vi "Extraction - Create index file.vi"(8 "Error In":errorcluster, 9 "Data":string[][](array[string]), 10 "Heading":string[](array[string]), 11 "report file path":path) -> (0 "Error Out":errorcluster)   [LabVIEW 2020]
uses:
  <vilib>/Utility/NIReport.llb/Append Text Table to Report (wrap).vi
  <vilib>/Utility/NIReport.llb/NI_report.lvclass
  <vilib>/Utility/NIReport.llb/Excel/NI_Excel.lvclass
panel:
  out "stripped path":path
  in  "save":bool=TRUE
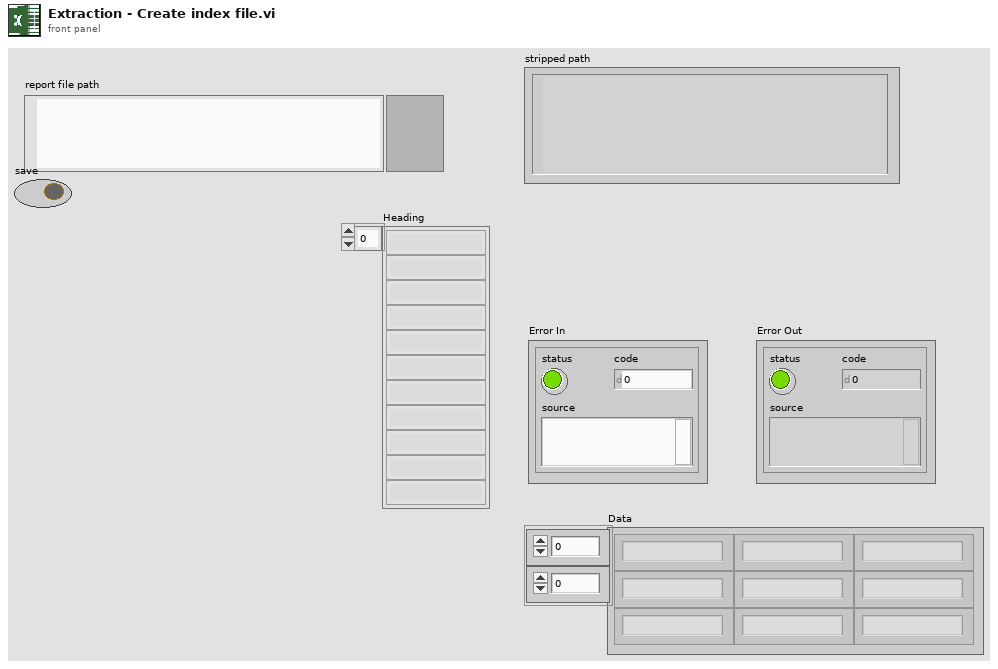
[diagram p1: front panel]
types:
  T1 = enum32{"invalid app kind", "Development System", "Run Time System", "Student Edition", "Embedded LabVIEW", "Evaluation", "Custom"}
  T2 = cluster{"position (excel)":cluster{"row":i32, "column":i32}, "name (excel)":string, "bookmark (word)":string}
  T3 = enum16{"Standard Report", "HTML", "Word", "Excel"}
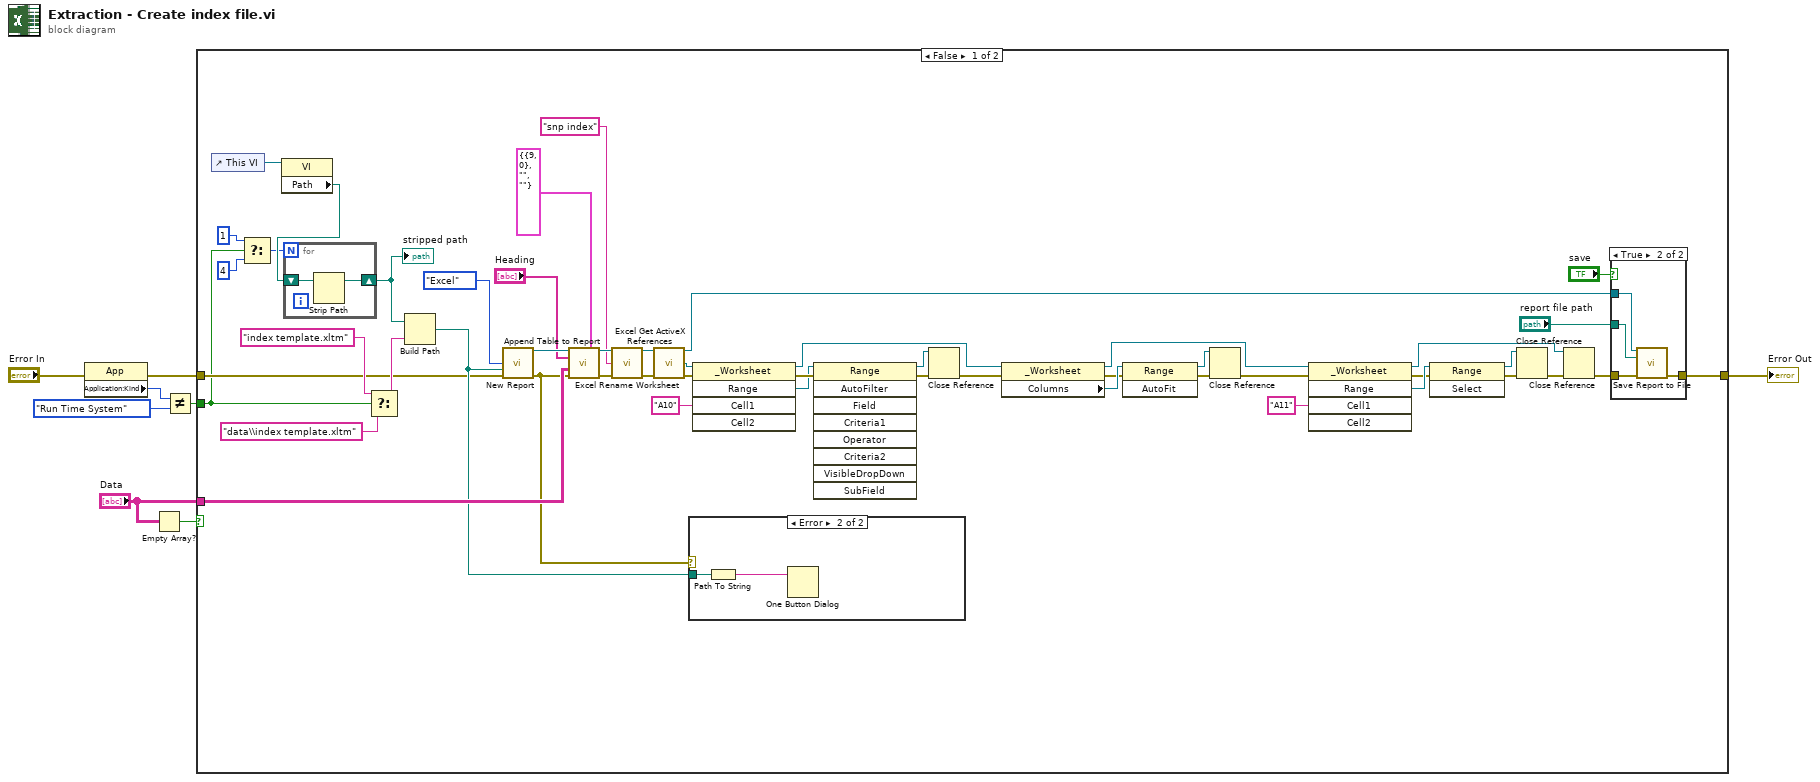
[diagram p0: block diagram]
diagram:
  n1 = property on="Property Node" class="App"(error in="Error In") -> (error out=w3:errorcluster, "Application:Kind"=w2:T1)  [unwired: 1 in, 1 out]
  n2 = Empty Array?(array="Data") -> (empty?=w5:bool)
  n3 = Not Equal?(x=w2, y=T1."Run Time System") -> (x != y?=w1:bool)
  n4 = case shown="False" w5 {
    tunnel: [w52 w68] -> w7
    tunnel: "Data" -> [w26 _]
    tunnel: w3 -> [w11 w68]
    tunnel: w1 -> [w10 _]
    frame False {
      n5 = control-ref of="This VI"() -> (w19:refnum<vi>)
      n6 = Select(t=1, s=w10, f=4) -> (s? t:f=w14:i32)
      n7 = property class="VI"(reference=w19) -> ("Path"=w28:path)  [unwired: 1 in, 2 out]
      n8 = for {
        N: w14 -> [_]
        shift-right: [w61] -> w27
        shift-left: w28 -> [w62]
        n9 = Strip Path(path=w62) -> (stripped path=w61:path)  [unwired: 1 out]
      }
      "stripped path" <- w27
      n10 = Select(t="index template.xltm" ("name or relative path"), s=w10, f="data\\index template.xltm" ("name or relative path")) -> (s? t:f=w16:string)
      n11 = Build Path(base path=w27, name or relative path=w16) -> (appended path=w15:path)
      n12 = call <vilib>:"New Report.vi"("report type"=T3."Excel", "template (empty)"=w15, "error in (no error)"=w11) -> ("report out"=w57:refnum<class "NI_report.lvclass">, "error out"=w9:errorcluster)  [unwired: 11 in]
      n13 = call-poly <vilib>:"Append Table to Report.vi"("report in"=w57, "MS Office parameters"=T2 {"position (excel)"={"row"=9, "column"=0}, "name (excel)"="", "bookmark (word)"=""}, "column headers"="Heading", "text data"=w26, "error in (no error)"=w9) -> ("report out"=w50:refnum<class "NI_report.lvclass">, "error out"=w51:errorcluster)  [unwired: 7 in, 2 out]
      n14 = call <vilib>:"Excel Rename Worksheet.vi"("report in"=w50, "worksheet name (\"\")"="snp index" ("worksheet name (\"\")"), "error in (no error)"=w51) -> ("report out"=w49:refnum<class "NI_report.lvclass">, "error out"=w48:errorcluster)  [unwired: 11 in]
      n15 = call <vilib>:"Excel Get ActiveX References.vi"("report in"=w49, "error in (no error)"=w48) -> ("report out"=w47:refnum<class "NI_report.lvclass">, "Excel._Worksheet"=w25:refnum<k7>, "error out"=w24:errorcluster)  [unwired: 7 in, 4 out]
      n16 = case shown="Error" w9 {
        tunnel: w15 -> [_ w60]
        frame No Error {
        }
        frame Error {
          n17 = Path To String(path=w60) -> (string=w59:string)
          n18 = One Button Dialog(message=w59) -> ()  [unwired: 1 in, 1 out]
        }
      }
      n19 = invoke class="_Worksheet" method="Range"(reference=w25, error in=w24, "Cell1"="A10") -> (reference out=w23:refnum<k7>, error out=w43:errorcluster, "Range"=w42:refnum<k7>)  [unwired: 2 in, 2 out]
      n20 = invoke class="Range" method="AutoFilter"(reference=w42, error in=w43) -> (reference out=w36:refnum<k7>, error out=w29:errorcluster)  [unwired: 7 in, 7 out]
      n21 = Close Reference(reference=w36, error in (no error)=w29) -> (error out=w21:errorcluster)
      n22 = property class="_Worksheet"(reference=w23, error in=w21) -> (reference out=w22:refnum<k7>, error out=w41:errorcluster, "Columns"=w44:refnum<k7>)
      n23 = invoke class="Range" method="AutoFit"(reference=w44, error in=w41) -> (reference out=w37:refnum<k7>, error out=w34:errorcluster)  [unwired: 1 in, 1 out]
      n24 = Close Reference(reference=w37, error in (no error)=w34) -> (error out=w20:errorcluster)
      n25 = invoke class="_Worksheet" method="Range"(reference=w22, error in=w20, "Cell1"="A11") -> (reference out=w33:refnum<k7>, error out=w39:errorcluster, "Range"=w40:refnum<k7>)  [unwired: 2 in, 2 out]
      n26 = invoke class="Range" method="Select"(reference=w40, error in=w39) -> (reference out=w35:refnum<k7>, error out=w30:errorcluster)  [unwired: 1 in, 1 out]
      n27 = Close Reference(reference=w35, error in (no error)=w30) -> (error out=w32:errorcluster)
      n28 = Close Reference(reference=w33, error in (no error)=w32) -> (error out=w31:errorcluster)
      n29 = case shown="True" "save" {
        tunnel: w47 -> [_ w67]
        tunnel: "report file path" -> [_ w66]
        tunnel: [w63 w65] -> w52
        tunnel: w31 -> [w63 w64]
        frame False {
        }
        frame True {
          n30 = call-dynamic "Save Report to File.vi"("report in"=w67, "report file path"=w66, "error in (no error)"=w64) -> ("error out"=w65:errorcluster)  [unwired: 11 in, 1 out]
        }
      }
    }
    frame True {
    }
  }
  "Error Out" <- w7
